vi "Assert Not Error.vi"(4 "Execution time (s)":dbl=-1.0, 6 "error code (1)":i32=1, 7 "Label":string, 8 "error in":errorcluster, 11 "error":errorcluster) -> (0 "error out":errorcluster, 2 "Properties":refnum<class "Properties.Assert.lvclass">)   [LabVIEW 2021, in "Bananas.lvlib"]
uses:
  Bananas.lvlib
  <vilib>/addons/_JKI Toolkits/Caraya/classes/Properties.Assert/Properties.Assert.lvclass
  Banana/Banana.lvclass/Banana.ctl
  AssetError/AssertError.lvclass/AssertError.ctl
  AssetError/Write Error.vi
  AssetError/Write Not_.vi
  <vilib>/LabVIEW Open Source Project/Data Manipulation/Variant/Variant_SetName.vi
  <vilib>/LabVIEW Open Source Project/Data Manipulation/Variant/Variant_BuildClusterFromElementArray.vi
  <vilib>/LabVIEW Open Source Project/Data Manipulation/Variant/Variant_EmptyCluster.vi
  AssetError/AssertError.lvclass
  C:/Repositories/LVOS/Bananas/lv-src/Bananas/BananaPeel/BananaPeel.lvclass
  <vilib>/LabVIEW Open Source Project/Data Manipulation/Variant/Variant_ListElements.vi
  <vilib>/LabVIEW Open Source Project/Data Manipulation/TypeDescriptor/TypeDescriptor_SetName.vi
  <vilib>/Utility/GetType.llb/TD_Create Cluster.vi
  AssertTrue/AssertTrue.lvclass
  AssertFalse/AssertFalse.lvclass
  AssertEqualValue/AssertEqualValue.lvclass
  AssertEqualType/AssertEqualType.lvclass
  AssertCompareValue/AssertCompareValue.lvclass
  AssertAlmostEqual/AssertAlmostEqualValue.lvclass
  <vilib>/addons/_JKI Toolkits/Caraya/classes/Assert/Assert.lvclass
  Banana/Banana.lvclass
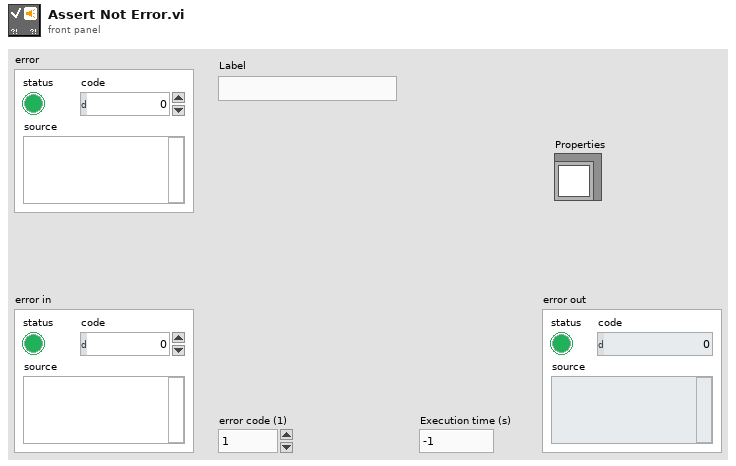
[diagram p1: front panel]
types:
  T1 = typedef "Bananas.lvlib/Assertion Strategies -- cluster.ctl" = cluster{"AssertTrue":refnum<class "AssertTrue.lvclass">, "AssertFalse":refnum<class "AssertFalse.lvclass">, "AssertEqualValue":refnum<class "AssertEqualValue.lvclass">, "AssertEqualType":refnum<class "AssertEqualType.lvclass">, "AssertCompareValue":refnum<class "AssertCompareValue.lvclass">, "AssertError":refnum<class "AssertError.lvclass">, "AssertAlmostEqual":refnum<class "AssertAlmostEqualValue.lvclass">}
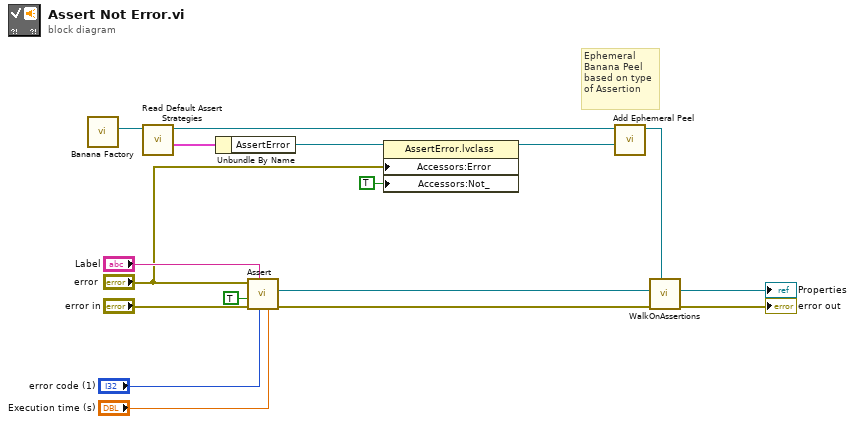
[diagram p0: block diagram]
diagram:
  # "Ephemeral\nBanana Peel\nbased on type\nof Assertion"
  n1 = call "Banana Factory.vi"() -> ("Bunch"=w7:refnum<class "Banana.lvclass">)  [unwired: 10 in, 1 out]
  n2 = call "Read Default Assert Strategies.vi"("Banana in"=w7) -> ("Strategies"=w5:T1, "Banana out"=w6:refnum<class "Banana.lvclass">)  [unwired: 9 in]
  n3 = Unbundle By Name(w5) -> ("AssertError"=w3:refnum<class "AssertError.lvclass">)
  n4 = call-poly <vilib>:"Assert.vi"("Execution time (s)"="Execution time (s)", "error code (1)"="error code (1)", "Label"="Label", "error in (no error)"="error in", "Register with caller test (F)"=TRUE, "Not Error?"="error") -> ("error out"=w12:errorcluster, "Properties.Assert"=w10:refnum<class "Properties.Assert.lvclass">)  [unwired: 4 in]
  n5 = property class="AssertError.lvclass"(reference=w3, "Accessors:Error"="error", "Accessors:Not_"=TRUE ("Not_")) -> (reference out=w2:refnum<class "AssertError.lvclass">)  [unwired: 1 in, 1 out]
  n6 = call "Add Ephemeral Peel.vi"("BananaPeel"=w2, "Bunch"=w6) -> ("Bunch"=w8:refnum<class "Banana.lvclass">)  [unwired: 9 in]
  n7 = call "WalkOnAssertions.vi"("Bunch"=w8, "error in (no error)"=w12, "Properties"=w10) -> ("error out"=→"error out":errorcluster, "Properties out"=→"Properties":refnum<class "Properties.Assert.lvclass">)  [unwired: 7 in]
